vi "[BLE Test] ble_read_write_characteristics (old).vi"() -> ()   [LabVIEW 2015]
uses:
  Lib_Bled112 toolkit/type_def/connection_status_bundle.ctl
  Lib_Bled112 toolkit/type_def/address_type.ctl
  Lib_Bled112 toolkit/ble_functions/ble_write_by_service_characteristic_uint8array.vi
  Lib_Bled112 toolkit/ble_functions/ble_write_by_handle_uint8array.vi
panel:
  out "Scan success?":bool
  out "BLED112 Dongle Info":string="Major: 1, Minor: 3, Patch: 2, Build: 122, LL ver: 3, Protocol ver: 1 and HW ver: 3  "
  out "그래프 타이머 값 1":u32=9582380
  out "CDC(PCAP02) Graph":waveform(sgl)[](graph)=[{"t0"=timestamp(3554331896.4574084 s since 1904-01-01), "dt"=0.03, "Y"=[1.0007696]}, {"t0"=timestamp(3554331896.4574084 s since 1904-01-01), "dt"=0.03, "Y"=[1.0004687]}]
  out "Working Time(H:M:S)":string="00:01:58"
  out "ms 타이머 값 2":u32=9464045
  out "Get Device name":bool
  out "Get handle table":bool
  in  "Device List":i32(listbox)=2
  out "Rx packet Interval graph":u32(graph)=30
  in  "Program Exit":bool=TRUE
  in  "Set-Interval":bool
  out "Rx 2":bool=TRUE
  out "부분배열 2":u8[](array[numeric])=[253, 79, 255, 49, 255, 79, 255, 60, 255, 209, 65, 123, 0, 0, 0, 0, 0, 0, 0, 0] format="%x"
  out "Data-IMU":dbl=-3.014375 format="%.10f"
  out "Hex-IMU":i16=-689 format="%x"
  out "웨이브폼 차트-IMU":dbl(graph)=-3.014375
  in  "Index-IMU ch.":u8(slide)=1 min=1 max=6 step=1 scale=1.0..6.0
  out "Rx 문자열 2":string
  out "IMU-Rx time(ms)":u32=15
  out "IMU Rx OK":bool=TRUE
  out "CDC Rx OK":bool=TRUE
  out "CDC-Rx time(ms)":u32=15
  out "ms 타이머 값":u32=9582439
  out "Entire-Rx time(ms)":i32=30
  in  "Index-CDC ch.":u8(slide)=1 min=1 max=6 step=1 scale=1.0..6.0
  out "웨이브폼 차트 - CDC":sgl(graph)=1.0007696
  out "Hex-CDC":u32=2098766 format="%x"
  out "Data-CDC":dbl=1.0007696151733398 format="%.10f"
  out "부분배열":u8[](array[numeric])=[32, 6, 78, 32, 3, 215, 32, 6, 110, 32, 71, 249, 32, 115, 92, 32, 30, 38, 1, 0] format="%x"
  out "Rx 1":bool=TRUE
  in  "Tx 문자열":string="\nBLED112 Test\n"
  in  "Tx Send":bool
  out "Rx Cnt":i32=3775
  in  "Rx Stop":bool=TRUE
  out "Rx 문자열 1":string
  out "Connected":bool
  out "Device Name":string
  out "Address Type":enum16{"Public", "Random"}(ring)=enum."Random"
  out "Handle table":string[][](array[string])
  out "Connection Status":T1 {"Address Type" items=["Public", "Random"]}
  out "Scanning":bool
  in  "Device Connect":bool=TRUE
  out "MAC Address":string="D9:2F:10:92:34:F2"
  in  "COM Bluegiga in":refnum<visa-resource-name>="COM8"
  # "GEN4 1st PP - BLE(Bluetooth Low Energy) Test"
  # "CDC Data"
  # "SCAN"
  # "DEVICES FOUND"
  # "CONNECT"
  # "Introduce the MAC Address and Address Type of the device you want to connect and click in the CONTINUE button"
  # "IMU Data"
  # "Service 0x1800\nCharacteristic 0x2A00\nDevice Name"
  # "READING DEVICE NAME"
  # "Read"
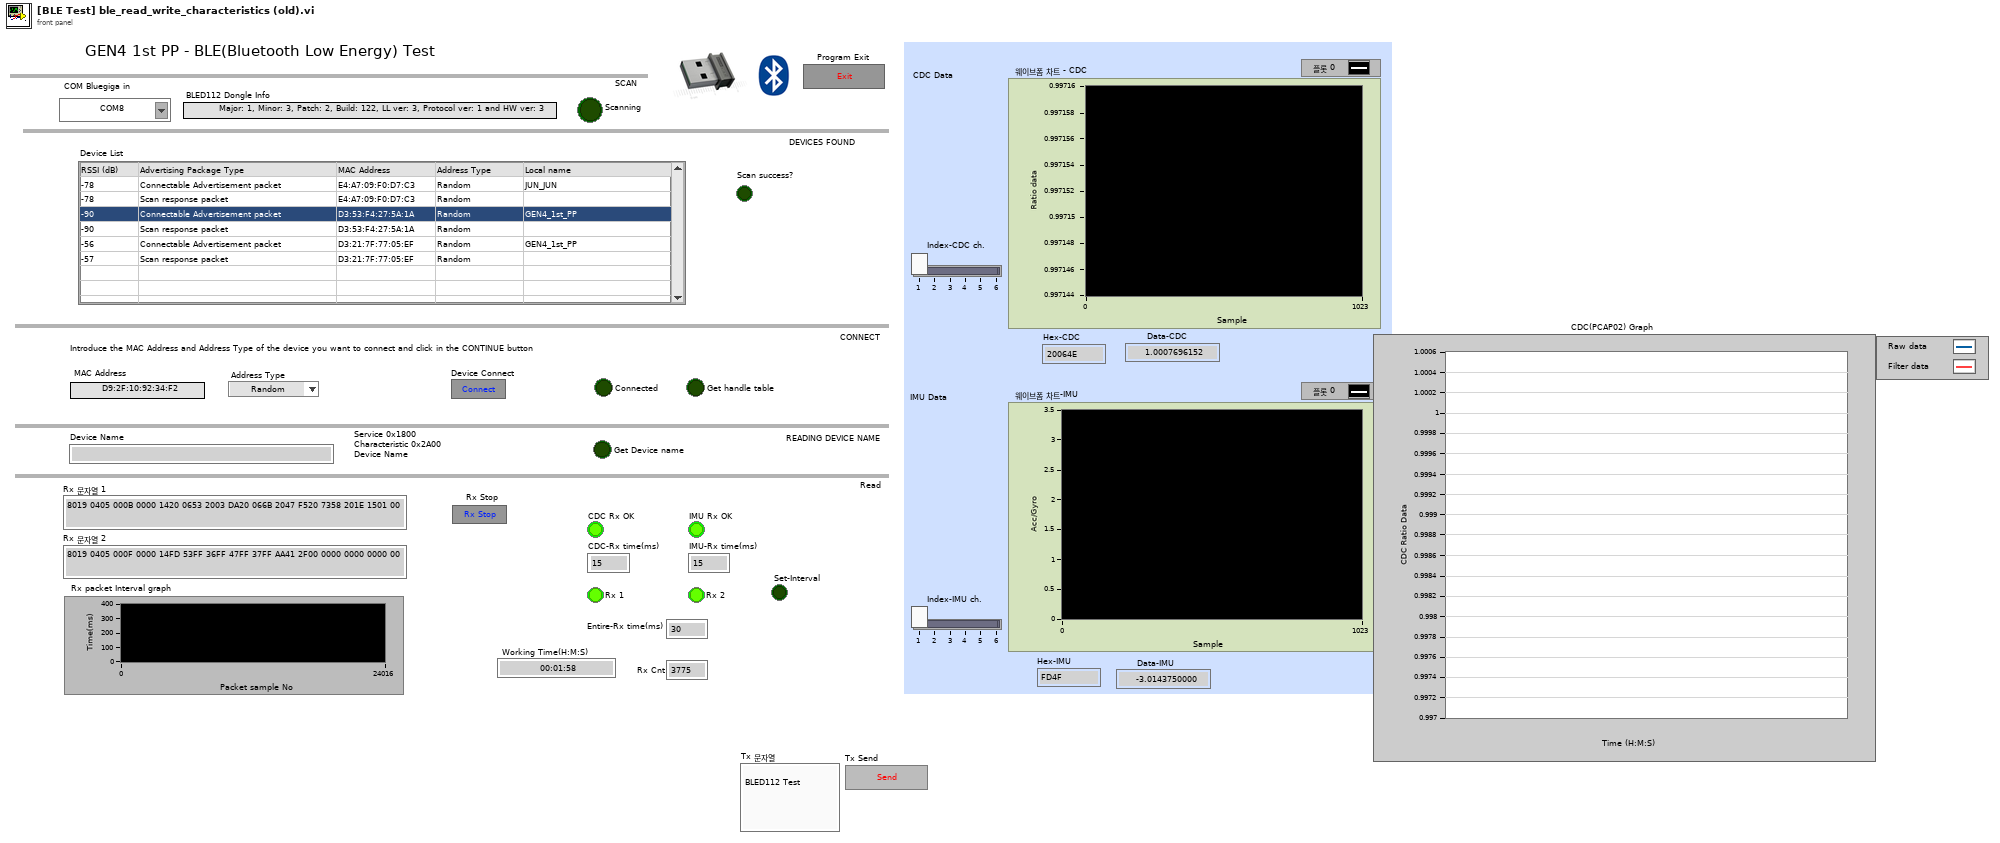
[diagram p1: front panel]
types:
  T1 = typedef "connection_status_bundle.ctl" = cluster{"MAC Address":string, "cnx handle":u8, "cnx flags":u8, "Address Type":T2, "Connection Interval (ms)":u16, "Timeout(ms)":u16, "Latency":u16, "bonding handle":u8}
  T2 = typedef "address_type.ctl" = u8
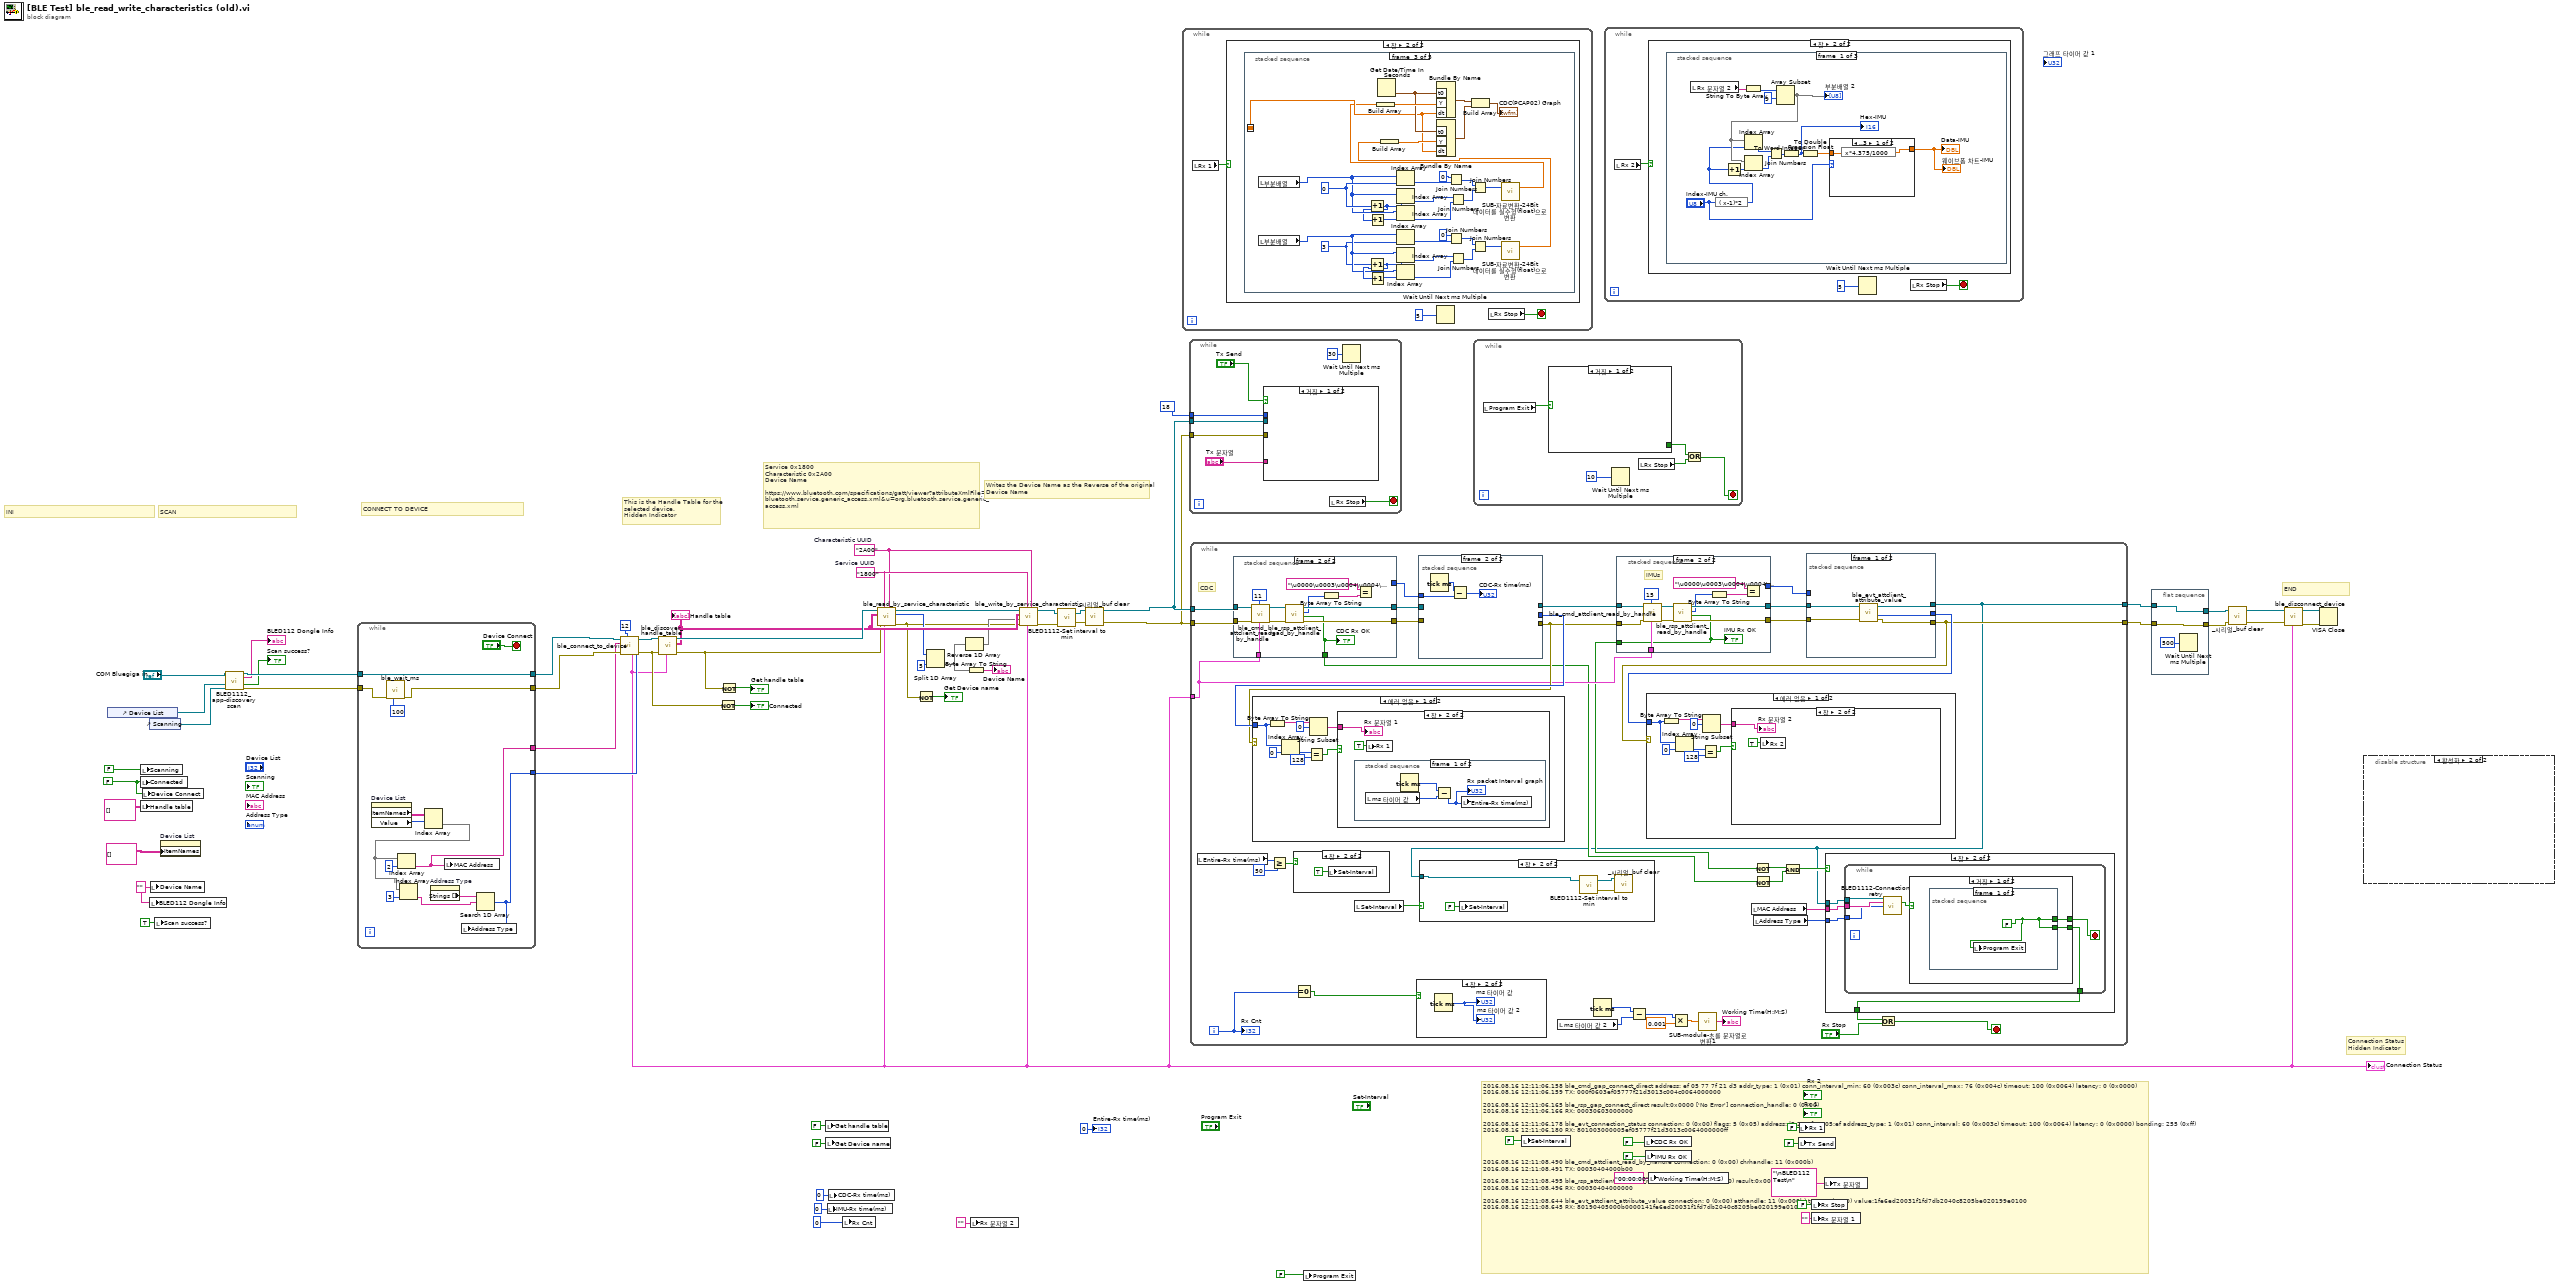
[diagram p0: block diagram]
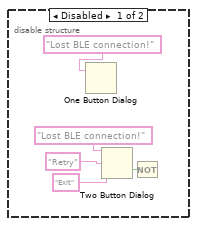
[diagram p2: hidden frame]
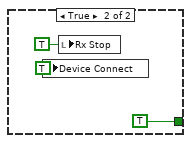
[diagram p3: hidden frame]
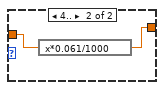
[diagram p5: hidden frame]
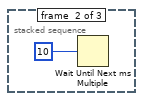
[diagram p6: hidden frame]
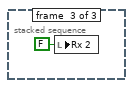
[diagram p7: hidden frame]
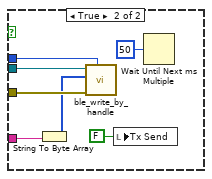
[diagram p8: hidden frame]
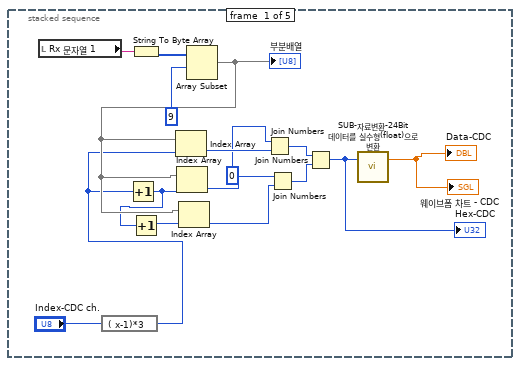
[diagram p10: hidden frame]
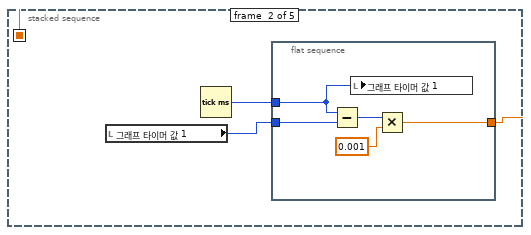
[diagram p11: hidden frame]
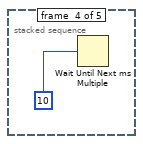
[diagram p12: hidden frame]
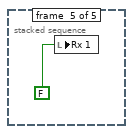
[diagram p13: hidden frame]
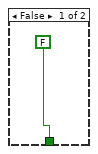
[diagram p16: hidden frame]
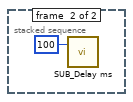
[diagram p17: hidden frame]
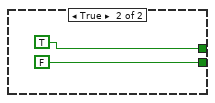
[diagram p18: hidden frame]
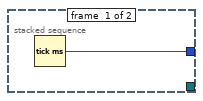
[diagram p20: hidden frame]
diagram:
  w50 = "2A00"  # Characteristic UUID
  w51 = "1800"  # Service UUID
  w4 = "" ("Device Name")
  w61 = FALSE ("Connected")
  # "2016.08.16 12:11:06.158 ble_cmd_gap_connect_direct address: ef 05 77 7f 21 d3 addr_type: 1 (0x01) conn_interval_min: 60 (0x003c) conn_interval_max: 76 (0x004c) timeout: 100 (0x0064) latency: 0 (0x0000)\n2016.08.16 12:11:06.159 TX: 000f0603ef05777f21d3013c004c0064000000\n\n2016.08.16 12:11:06.165 ble_rsp_gap_connect_direct result:0x0000 ['No Error'] connection_handle: 0 (0x00)\n2016.08.16 12:11:06.166 RX: 00030603000000\n\n2016.08.16 12:11:06.178 ble_evt_connection_status connection: 0 (0x00) flags: 5 (0x05) address:d3:21:7f:77:05:ef address_type: 1 (0x01) conn_interval: 60 (0x003c) timeout: 100 (0x0064) latency: 0 (0x0000) bonding: 255 (0xff)\n2016.08.16 12:11:06.180 RX: 801003000005ef05777f21d3013c0064000000ff\n\n\n\n\n2016.08.16 12:11:08.490 ble_cmd_attclient_read_by_handle connection: 0 (0x00) chrhandle: 11 (0x000b)\n2016.08.16 12:11:08.491 TX: 00030404000b00\n\n2016.08.16 12:11:08.495 ble_rsp_attclient_read_by_handle connection: 0 (0x00) result:0x0000 ['No Error']\n2016.08.16 12:11:08.496 RX: 00030404000000\n\n2016.08.16 12:11:08.644 ble_evt_attclient_attribute_value connection: 0 (0x00) atthandle: 11 (0x000b) type: 0 (0x00) value:1fe6ed20031f1fd7db2040c8205be020199e0100\n2016.08.16 12:11:08.645 RX: 80190405000b0000141fe6ed20031f1fd7db2040c8205be020199e0100"
  # "Writes the Device Name as the Reverse of the original\nDevice Name"
  # "Service 0x1800\nCharacteristic 0x2A00\nDevice Name\n\nhttps://www.bluetooth.com/specifications/gatt/viewer?attributeXmlFile=org.bluetooth.service.generic_access.xml&u=org.bluetooth.service.generic_access.xml"
  # "This is the Handle Table for the\nselected device. \nHidden Indicator"
  # "Connection Status\nHidden Indicator"
  # "CONNECT TO DEVICE"
  # "SCAN"
  # "END"
  # "INI"
  n1 = control-ref of="Device List"() -> (w8:refnum<vi>)
  n2 = local write "Connected"(w61) -> ()
  n3 = local write "Handle table"(string[][] [] ("Handle table")) -> ()
  n4 = local write "Scanning"(FALSE ("Scanning")) -> ()
  n5 = local write "Device Connect"(w61) -> ()
  n6 = control-ref of="Scanning"() -> (w7:refnum<vi>)
  n7 = local write "BLED112 Dongle Info"(w4) -> ()
  n8 = local write "Device Name"(w4) -> ()
  n9 = local write "Scan success?"(TRUE ("Scan success?")) -> ()
  n10 = property on="Device List" class="MCListbox (엄격한)"("ItemNames"=string[][] [] ("Devices")) -> ()  [unwired: 2 in, 2 out]
  n11 = call "BLED1112_app-discovery scan.vi"("COM in"="COM Bluegiga in", "Device List"=w8, "LED ref"=w7) -> ("COM out"=w6:refnum<visa-resource-name>, "BLED112 Dongle Info"=→"BLED112 Dongle Info":string, "Scan success?"=→"Scan success?":bool, "error out"=w3:errorcluster)  [unwired: 8 in, 1 out]
  n12 = while {
    tunnel: w3 -> [w81]
    tunnel: [w80] -> w68
    tunnel: w6 -> [w80]
    tunnel: [w79] -> w67
    tunnel: [w74] -> w64
    tunnel: [w69] -> w63
    stop <- "Device Connect" stop-if-true
    n13 = property on="Device List" class="MCListbox (엄격한)"() -> ("ItemNames"=w77:string[][], "Value"=w76:i32)  [unwired: 2 in, 2 out]
    n14 = call "ble_wait_ms.vi"("milliseconds to wait (100)"=u32 100, "error in (no error)"=w81) -> ("error out"=w79:errorcluster)  [unwired: 9 in]
    n15 = Index Array(array=w77, index (row)=w76) -> (element=w72:string[])  [unwired: 1 in]
    n16 = Index Array(array=w72, index=2 ("인덱스")) -> (element=w74:string)
    n17 = Index Array(array=w72, index=3 ("인덱스")) -> (element=w70:string)
    n18 = property on="Address Type" class="Enum (엄격한)"() -> ("Strings []"=w71:string[])  [unwired: 2 in, 2 out]
    n19 = local write "MAC Address"(w74) -> ()
    n20 = Search 1D Array(1D array=w71, element=w70) -> (index of element=w69:i32)  [unwired: 1 in]
    n21 = local write "Address Type"(w69) -> ()
  }
  n22 = call "ble_connect_to_device.vi"("Address Type"=w63, "Connection Interval Min (75ms)"=u16 12, "error in (no error)"=w67, "MAC Address"=w64, "COM Bluegiga in"=w68) -> ("error out"=w36:errorcluster, "COM Bluegiga out"=w38:refnum<visa-resource-name>, "Connection Status"=w14:T1)  [unwired: 4 in]
  "Connection Status" <- w14
  n23 = call "ble_discover_handle_table.vi"("Connection Status"=w14, "error in (no error)"=w36, "COM Bluegiga in"=w38) -> ("error out"=w35:errorcluster, "Handle table"=w49:string[][], "COM Bluegiga out"=w55:refnum<visa-resource-name>)  [unwired: 6 in]
  "Handle table" <- w49
  n24 = Not(x=w36) -> (.not. x?=→"Connected":bool)
  n25 = Not(x=w35) -> (.not. x?=→"Get handle table":bool)
  n26 = local write "Get handle table"(FALSE ("Get handle table")) -> ()
  n27 = local write "Get Device name"(FALSE ("Get Device name")) -> ()
  n28 = local write "IMU-Rx time(ms)"(u32 0 ("CDC-Rx time(ms)")) -> ()
  n29 = local write "CDC-Rx time(ms)"(u32 0 ("CDC-Rx time(ms)")) -> ()
  n30 = local write "Rx Cnt"(u32 0 ("CDC-Rx time(ms)")) -> ()
  n31 = call "ble_read_by_service_characteristic.vi"("Characteristic UUID"=w50, "Connection Status"=w14, "Service UUID"=w51, "error in (no error)"=w35, "Handle table"=w49, "COM Bluegiga in"=w55) -> ("error out"=w32:errorcluster, "characteristic value"=w48:u8[], "COM Bluegiga out"=w52:refnum<visa-resource-name>)  [unwired: 3 in]
  n32 = Not(x=w32) -> (.not. x?=→"Get Device name":bool)
  n33 = Split 1D Array(array=w48, index=5) -> (second subarray=w47:u8[])  [unwired: 1 out]
  n34 = Reverse 1D Array(array=w47) -> (reversed array=w46:u8[])
  n35 = Byte Array To String(unsigned byte array=w47) -> (string=→"Device Name":string)
  n36 = local write "Rx 문자열 2"("" ("Rx 문자열 2")) -> ()
  n37 = call-poly "ble_write_by_service_characteristic.vi"("Characteristic UUID"=w50, "Connection Status"=w14, "Service UUID"=w51, "error in (no error)"=w32, "data"=w46, "Handle table"=w49, "COM Bluegiga in"=w52) -> ("error out"=w24:errorcluster, "COM Bluegiga out"=w25:refnum<visa-resource-name>)  [unwired: 3 in]
  n38 = call "BLED1112-Set interval to min.vi"("에러 입력(에러 없음)"=w24, "VISA 리소스 이름"=w25) -> ("에러 출력"=w22:errorcluster, "VISA 리소스 이름 출력"=w23:refnum<visa-resource-name>)
  n39 = call "_시리얼_buf clear.vi"("에러 출력 2"=w22, "시리얼 포트"=w23) -> ("에러 출력"=w43:errorcluster, "시리얼 포트 2"=w44:refnum<visa-resource-name>)  [unwired: 2 in]
  n40 = while {
    stop <- w85 stop-if-true
    n41 = local read "Rx 1"() -> (w84:bool)
    n42 = case shown="참" w84 {
      frame False {
      }
      frame True {
        n43 = stacked-sequence {
          seq-local: [_ w102 _ _ _] -> [_ _ w134 _ _]
          frame #0 {
            n44 = local read "Rx 문자열 1"() -> (w101:string)
            n45 = expression code="( x-1)*3"("Index-CDC ch.") -> (w88:u8)
            n46 = Increment(x=w88) -> (x+1=w87:u8)
            n47 = String To Byte Array(string=w101) -> (unsigned byte array=w100:u8[])
            n48 = Increment(x=w87) -> (x+1=w86:u8)
            n49 = Array Subset(array=w100, index=9 ("인덱스")) -> (w98:u8[])  [unwired: 1 in]
            "부분배열" <- w98
            n50 = Index Array(array=w98, index=w88) -> (element=w95:u8)
            n51 = Index Array(array=w98, index=w87) -> (element=w96:u8)
            n52 = Index Array(array=w98, index=w86) -> (element=w97:u8)
            n53 = Join Numbers(hi=u8 0 ("인덱스"), lo=w95) -> ((hi.lo)=w92:u16)
            n54 = Join Numbers(hi=w96, lo=w97) -> ((hi.lo)=w93:u16)
            n55 = Join Numbers(hi=w92, lo=w93) -> ((hi.lo)=w91:u32)
            "Hex-CDC" <- w91
            n56 = call "SUB-자료변환-24Bit 데이터를 실수형(float)으로 변환.vi"("U32"=w91) -> ("FP32"=→"Data-CDC" →"웨이브폼 차트 - CDC":sgl)  [unwired: 2 in]
          }
          frame #1 {
            n57 = local read "그래프 타이머 값 1"() -> (w104:u32)
            n58 = Tick Count (ms)() -> (millisecond timer value=w103:u32)
            n59 = flat-sequence {
              tunnel: w103 -> [w109]
              tunnel: w104 -> [w106]
              tunnel: [w105] -> w102
              frame #0 {
                n60 = Subtract(x=w109, y=w106) -> (x-y=w107:u32)
                n61 = local write "그래프 타이머 값 1"(w109) -> ()
                n62 = Multiply(x=w107, y=0.001 ("dt")) -> (x*y=w105:dbl)
              }
            }
          }
          frame #2 {
            w112 = u8 3 ("인덱스")
            w133 = u8 0 ("인덱스")
            n63 = local read "부분배열"() -> (w132:u8[])
            n64 = local read "부분배열"() -> (w113:u8[])
            n65 = Increment(x=w133) -> (x+1=w124:u8)
            n66 = Increment(x=w112) -> (x+1=w121:u8)
            n67 = Increment(x=w124) -> (x+1=w123:u8)
            n68 = Increment(x=w121) -> (x+1=w122:u8)
            n69 = Get Date/Time In Seconds() -> (seconds since 1Jan1904=w138:timestamp)
            n70 = Index Array(array=w132, index=w133) -> (element=w129:u8)
            n71 = Index Array(array=w113, index=w112) -> (element=w116:u8)
            n72 = Index Array(array=w132, index=w124) -> (element=w130:u8)
            n73 = Index Array(array=w132, index=w123) -> (element=w131:u8)
            n74 = Index Array(array=w113, index=w121) -> (element=w115:u8)
            n75 = Index Array(array=w113, index=w122) -> (element=w114:u8)
            n76 = Join Numbers(hi=u8 0 ("인덱스"), lo=w129) -> ((hi.lo)=w126:u16)
            n77 = Join Numbers(hi=u8 0 ("인덱스"), lo=w116) -> ((hi.lo)=w119:u16)
            n78 = Join Numbers(hi=w130, lo=w131) -> ((hi.lo)=w127:u16)
            n79 = Join Numbers(hi=w115, lo=w114) -> ((hi.lo)=w118:u16)
            n80 = Join Numbers(hi=w126, lo=w127) -> ((hi.lo)=w125:u32)
            n81 = Join Numbers(hi=w119, lo=w118) -> ((hi.lo)=w120:u32)
            n82 = call "SUB-자료변환-24Bit 데이터를 실수형(float)으로 변환.vi"("U32"=w125) -> ("FP32"=w111:sgl)  [unwired: 2 in]
            n83 = Build Array(w111) -> (w139:sgl[])
            n84 = Bundle By Name("t0"=w138, "Y"=w139, "dt"=w134) -> (w135:waveform(sgl))  [unwired: 1 in]
            n85 = call "SUB-자료변환-24Bit 데이터를 실수형(float)으로 변환.vi"("U32"=w120) -> ("FP32"=w110:sgl)  [unwired: 2 in]
            n86 = Build Array(w110) -> (w140:sgl[])
            n87 = Bundle By Name("t0"=w138, "Y"=w140, "dt"=w134) -> (w136:waveform(sgl))  [unwired: 1 in]
            n88 = Build Array(w135, w136) -> (→"CDC(PCAP02) Graph":waveform(sgl)[])
          }
          frame #3 {
            n89 = Wait Until Next ms Multiple(millisecond multiple=u32 10 ("ms 배수")) -> ()  [unwired: 1 out]
          }
          frame #4 {
            n90 = local write "Rx 1"(FALSE ("Rx")) -> ()
          }
        }
      }
    }
    n91 = Wait Until Next ms Multiple(millisecond multiple=u32 5 ("ms 배수")) -> ()  [unwired: 1 out]
    n92 = local read "Rx Stop"() -> (w85:bool)
  }
  n93 = while {
    tunnel: w44 -> [w146]
    tunnel: w43 -> [w145]
    tunnel: u16 18 ("Handle") -> [w144]
    stop <- w147 stop-if-true
    n94 = case shown="거짓" "Tx Send" {
      tunnel: w146 -> [_ w156]
      tunnel: w145 -> [_ w155]
      tunnel: w144 -> [_ w153]
      tunnel: "Tx 문자열" -> [_ w152]
      frame False {
      }
      frame True {
        n95 = String To Byte Array(string=w152) -> (unsigned byte array=w154:u8[])
        n96 = call-poly "ble_write_by_handle.vi"("Handle"=w153, "error in (no error)"=w155, "data (uint8array)"=w154, "COM Bluegiga in"=w156) -> ()  [unwired: 6 in, 2 out]
        n97 = local write "Tx Send"(FALSE ("Tx Send")) -> ()
        n98 = Wait Until Next ms Multiple(millisecond multiple=u32 50 ("ms 배수")) -> ()  [unwired: 1 out]
      }
    }
    n99 = local read "Rx Stop"() -> (w147:bool)
    n100 = Wait Until Next ms Multiple(millisecond multiple=u32 30 ("ms 배수")) -> ()  [unwired: 1 out]
  }
  n101 = while {
    tunnel: w44 -> [w190]
    tunnel: w43 -> [w189]
    tunnel: w14 -> [w184]
    tunnel: [w160] -> w59
    tunnel: [w182] -> w58
    i -> [w168]
    stop <- w176 stop-if-true
    # "CDC"
    n102 = local read "Entire-Rx time(ms)"() -> (w171:i32)
    n103 = stacked-sequence {
      tunnel: [_ w239] -> w192
      tunnel: [_ w238] -> w191
      tunnel: w190 -> [_ w237]
      tunnel: w189 -> [_ w236]
      tunnel: w184 -> [_ w235]
      tunnel: [w230 _] -> w181
      tunnel: [_ w231] -> w173
      frame #0 {
        n104 = Tick Count (ms)() -> (millisecond timer value=w230:u32)
      }
      frame #1 {
        n105 = call "ble_cmd_attclient_read_by_handle.vi"("Connection Status"=w235, "chrHandle"=u16 11 ("Handle"), "error in (no error)"=w236, "COM Bluegiga in"=w237) -> ("error out"=w240:errorcluster, "COM Bluegiga out"=w241:refnum<visa-resource-name>)  [unwired: 6 in]
        n106 = call "ble_rsp_attclient_read_by_handle.vi"("error in (no error)"=w240, "COM Bluegiga in"=w241) -> ("error out"=w239:errorcluster, "success?"=w231:bool, "full message package"=w232:u8[], "COM Bluegiga out"=w238:refnum<visa-resource-name>)  [unwired: 6 in]
        "CDC Rx OK" <- w231
        n107 = Byte Array To String(unsigned byte array=w232) -> (string=w233:string)
        n108 = Equal?(x="\u0000\u0003\u0004\u0004\u0000\u0000\u0000", y=w233) -> ()  [unwired: 1 out]
      }
    }
    n109 = Greater Or Equal?(x=w171, y=50) -> (x >= y?=w170:bool)
    n110 = case shown="참" w170 {
      frame False {
      }
      frame True {
        n111 = local write "Set-Interval"(TRUE ("Set-Interval")) -> ()
      }
    }
    n112 = Equal To 0?(x=w168) -> (x = 0?=w167:bool)
    n113 = local read "Set-Interval"() -> (w179:bool)
    n114 = case shown="참" w167 {
      frame False {
      }
      frame True {
        n115 = Tick Count (ms)() -> (millisecond timer value=→"ms 타이머 값" →"ms 타이머 값 2":u32)
      }
    }
    n116 = stacked-sequence {
      tunnel: [w263 _] -> w186
      tunnel: [w261 _] -> w193
      tunnel: [w262 _] -> w185
      tunnel: w192 -> [w265 _]
      tunnel: w191 -> [w264 _]
      tunnel: w181 -> [_ w267]
      frame #0 {
        n117 = call "ble_evt_attclient_attribute_value.vi"("error in (no error)"=w265, "COM Bluegiga in"=w264) -> ("error out"=w262:errorcluster, "full message package"=w261:u8[], "COM Bluegiga out"=w263:refnum<visa-resource-name>)  [unwired: 6 in, 1 out]
      }
      frame #1 {
        n118 = Tick Count (ms)() -> (millisecond timer value=w268:u32)
        n119 = Subtract(x=w268, y=w267) -> (x-y=→"CDC-Rx time(ms)":u32)
      }
    }
    n120 = case shown="에러 없음" w185 {
      tunnel: w193 -> [w274 _]
      frame No Error {
        n121 = Byte Array To String(unsigned byte array=w274) -> (string=w276:string)
        n122 = Index Array(array=w274, index=0 ("인덱스")) -> (element=w272:u8)
        n123 = Equal?(x=w272, y=u16 128 ("Handle")) -> (x = y?=w270:bool)
        n124 = String Subset(string=w276, offset (0)=0 ("오프셋(0)")) -> (substring=w269:string)  [unwired: 1 in]
        n125 = case shown="참" w270 {
          tunnel: w269 -> [_ w278]
          frame False {
          }
          frame True {
            n126 = stacked-sequence {
              frame #0 {
                n127 = local read "ms 타이머 값"() -> (w281:u32)
                n128 = Tick Count (ms)() -> (millisecond timer value=w280:u32)
                n129 = Subtract(x=w280, y=w281) -> (x-y=w279:u32)
                "Rx packet Interval graph" <- w279
                n130 = local write "Entire-Rx time(ms)"(w279) -> ()
              }
              frame #1 {
                n131 = Tick Count (ms)() -> (millisecond timer value=w282:u32)
                n132 = local write "ms 타이머 값"(w282) -> ()
              }
            }
            n133 = local write "Rx 1"(TRUE ("Rx")) -> ()
            "Rx 문자열 1" <- w278
          }
        }
      }
      frame Error {
      }
    }
    n134 = local read "ms 타이머 값 2"() -> (w165:u32)
    n135 = Tick Count (ms)() -> (millisecond timer value=w166:u32)
    n136 = stacked-sequence {
      tunnel: [_ w229] -> w188
      tunnel: [_ w228] -> w187
      tunnel: w186 -> [_ w224]
      tunnel: w185 -> [_ w223]
      tunnel: w184 -> [_ w222]
      tunnel: [w217 _] -> w180
      tunnel: [_ w218] -> w172
      frame #0 {
        n137 = Tick Count (ms)() -> (millisecond timer value=w217:u32)
      }
      frame #1 {
        # "IMUs"
        n138 = call "ble_cmd_attclient_read_by_handle.vi"("Connection Status"=w222, "chrHandle"=u16 15 ("Handle"), "error in (no error)"=w223, "COM Bluegiga in"=w224) -> ("error out"=w227:errorcluster, "COM Bluegiga out"=w226:refnum<visa-resource-name>)  [unwired: 6 in]
        n139 = call "ble_rsp_attclient_read_by_handle.vi"("error in (no error)"=w227, "COM Bluegiga in"=w226) -> ("error out"=w228:errorcluster, "success?"=w218:bool, "full message package"=w219:u8[], "COM Bluegiga out"=w229:refnum<visa-resource-name>)  [unwired: 6 in]
        "IMU Rx OK" <- w218
        n140 = Byte Array To String(unsigned byte array=w219) -> (string=w220:string)
        n141 = Equal?(x="\u0000\u0003\u0004\u0004\u0000\u0000\u0000", y=w220) -> ()  [unwired: 1 out]
      }
    }
    n142 = Subtract(x=w166, y=w165) -> (x-y=w162:u32)
    n143 = Multiply(x=w162, y=0.001) -> (x*y=w164:dbl)
    n144 = call "SUB-module-초를 문자열로 변환1.vi"("입력-초단위"=w164) -> ("시:분:초"=→"Working Time(H:M:S)":string)
    n145 = local read "MAC Address"() -> (w158:string)
    n146 = local read "Address Type"() -> (w157:enum16{"Public", "Random"})
    n147 = Not(x=w172) -> (.not. x?=w174:bool)
    n148 = Not(x=w173) -> (.not. x?=w175:bool)
    n149 = And(x=w174, y=w175) -> (x .and. y?=w177:bool)
    n150 = stacked-sequence {
      tunnel: [w255 _] -> w160
      tunnel: [w253 _] -> w183
      tunnel: [w254 _] -> w182
      tunnel: w187 -> [w257 _]
      tunnel: w188 -> [w256 _]
      tunnel: w180 -> [_ w259]
      frame #0 {
        n151 = call "ble_evt_attclient_attribute_value.vi"("error in (no error)"=w257, "COM Bluegiga in"=w256) -> ("error out"=w254:errorcluster, "full message package"=w253:u8[], "COM Bluegiga out"=w255:refnum<visa-resource-name>)  [unwired: 6 in, 1 out]
      }
      frame #1 {
        n152 = Tick Count (ms)() -> (millisecond timer value=w260:u32)
        n153 = Subtract(x=w260, y=w259) -> (x-y=→"IMU-Rx time(ms)":u32)
      }
    }
    n154 = case shown="참" w179 {
      tunnel: w160 -> [_ w213]
      frame False {
      }
      frame True {
        n155 = local write "Set-Interval"(FALSE ("Set-Interval")) -> ()
        n156 = call "BLED1112-Set interval to min.vi"("VISA 리소스 이름"=w213) -> ("에러 출력"=w214:errorcluster, "VISA 리소스 이름 출력"=w215:refnum<visa-resource-name>)  [unwired: 1 in]
        n157 = call "_시리얼_buf clear.vi"("에러 출력 2"=w214, "시리얼 포트"=w215) -> ()  [unwired: 2 in, 2 out]
      }
    }
    n158 = case shown="에러 없음" w182 {
      tunnel: w183 -> [w248 _]
      frame No Error {
        n159 = Byte Array To String(unsigned byte array=w248) -> (string=w250:string)
        n160 = Index Array(array=w248, index=0 ("인덱스")) -> (element=w246:u8)
        n161 = Equal?(x=w246, y=u16 128 ("Handle")) -> (x = y?=w244:bool)
        n162 = String Subset(string=w250, offset (0)=0 ("오프셋(0)")) -> (substring=w243:string)  [unwired: 1 in]
        n163 = case shown="참" w244 {
          tunnel: w243 -> [_ w252]
          frame False {
          }
          frame True {
            n164 = local write "Rx 2"(TRUE ("Rx")) -> ()
            "Rx 문자열 2" <- w252
          }
        }
      }
      frame Error {
      }
    }
    n165 = case shown="참" w177 {
      tunnel: w160 -> [_ w200]
      tunnel: [FALSE w197] -> w159
      tunnel: w158 -> [_ w199]
      tunnel: w157 -> [_ w198]
      frame False {
      }
      frame True {
        n166 = while {
          tunnel: w200 -> [w206]
          tunnel: w199 -> [w205]
          tunnel: w198 -> [w204]
          tunnel: [w201] -> w197
          stop <- w202 stop-if-true
          n167 = call "BLED1112-Connection retry.vi"("VISA 리소스 이름"=w206, "MAC Address"=w205, "Address Type"=w204) -> ("Connected"=w203:bool)  [unwired: 10 in, 2 out]
          n168 = case shown="거짓" w203 {
            tunnel: [w208 TRUE] -> w202
            tunnel: [w207 FALSE] -> w201
            frame False {
              n169 = stacked-sequence {
                tunnel: [w209 _] -> w208
                tunnel: [w209 _] -> w207
                frame #0 {
                  w209 = FALSE
                  n170 = local write "Program Exit"(w209) -> ()
                }
                frame #1 {
                  n171 = call "SUB_Delay ms.vi"("delay(ms)"=u32 100) -> ()  [unwired: 3 in]
                }
              }
            }
            frame True {
            }
          }
        }
      }
    }
    n172 = Or(x=w159, y="Rx Stop") -> (x .or. y?=w176:bool)
    "Rx Cnt" <- w168
  }
  n173 = local write "Program Exit"(FALSE ("정지")) -> ()
  n174 = while {
    stop <- w283 stop-if-true
    n175 = local read "Program Exit"() -> (w287:bool)
    n176 = case shown="거짓" w287 {
      tunnel: [_ TRUE] -> w284
      frame False {
      }
      frame True {
        n177 = local write "Device Connect"(TRUE ("Continue")) -> ()
        n178 = local write "Rx Stop"(TRUE ("Rx 정지")) -> ()
      }
    }
    n179 = Wait Until Next ms Multiple(millisecond multiple=u32 10 ("ms 배수")) -> ()  [unwired: 1 out]
    n180 = local read "Rx Stop"() -> (w285:bool)
    n181 = Or(x=w284, y=w285) -> (x .or. y?=w283:bool)
  }
  n182 = local write "Set-Interval"(FALSE ("Set-Interval")) -> ()
  n183 = while {
    stop <- w293 stop-if-true
    n184 = local read "Rx 2"() -> (w292:bool)
    n185 = case shown="참" w292 {
      frame False {
      }
      frame True {
        n186 = stacked-sequence {
          frame #0 {
            n187 = local read "Rx 문자열 2"() -> (w306:string)
            n188 = expression code="( x-1)*2"("Index-IMU ch.") -> (w297:u8)
            n189 = Increment(x=w297) -> (x+1=w296:u8)
            n190 = String To Byte Array(string=w306) -> (unsigned byte array=w305:u8[])
            n191 = Array Subset(array=w305, index=9 ("인덱스")) -> (w303:u8[])  [unwired: 1 in]
            "부분배열 2" <- w303
            n192 = Index Array(array=w303, index=w297) -> (element=w302:u8)
            n193 = Index Array(array=w303, index=w296) -> (element=w301:u8)
            n194 = Join Numbers(hi=w302, lo=w301) -> ((hi.lo)=w299:u16)
            n195 = To Word Integer(number=w299) -> (16bit integer=w295:i16)
            "Hex-IMU" <- w295
            n196 = To Double Precision Float(number=w295) -> (double precision float=w298:dbl)
            n197 = case shown="..3" "Index-IMU ch." {
              tunnel: [w308 w309] -> w300
              tunnel: w298 -> [w307 w310]
              frame ..3 {
                n198 = expression code="x*4.375/1000"(w307) -> (w308:dbl)
              }
              frame 4.. {
                n199 = expression code="x*0.061/1000"(w310) -> (w309:dbl)
              }
            }
            "Data-IMU" <- w300
            "웨이브폼 차트-IMU" <- w300
          }
          frame #1 {
            n200 = Wait Until Next ms Multiple(millisecond multiple=u32 10 ("ms 배수")) -> ()  [unwired: 1 out]
          }
          frame #2 {
            n201 = local write "Rx 2"(FALSE ("Rx")) -> ()
          }
        }
      }
    }
    n202 = Wait Until Next ms Multiple(millisecond multiple=u32 5 ("ms 배수")) -> ()  [unwired: 1 out]
    n203 = local read "Rx Stop"() -> (w293:bool)
  }
  n204 = local write "CDC Rx OK"(FALSE ("success?")) -> ()
  n205 = local write "IMU Rx OK"(FALSE ("success?")) -> ()
  n206 = local write "Working Time(H:M:S)"("00:00:00" ("Working Time(H:M:S)")) -> ()
  n207 = local write "Tx Send"(FALSE ("Tx Send")) -> ()
  n208 = local write "Rx 1"(FALSE ("Rx")) -> ()
  n209 = local write "Rx Stop"(FALSE ("Rx 정지")) -> ()
  n210 = local write "Rx 문자열 1"("" ("Rx 문자열")) -> ()
  n211 = local write "Tx 문자열"("\nBLED112 Test\n" ("Tx 문자열")) -> ()
  n212 = flat-sequence {
    tunnel: [w314] -> w13
    tunnel: w59 -> [w314]
    tunnel: [w313] -> w12
    tunnel: w58 -> [w313]
    frame #0 {
      n213 = Wait Until Next ms Multiple(millisecond multiple=u32 500 ("ms 배수")) -> ()  [unwired: 1 out]
    }
  }
  n214 = call "_시리얼_buf clear.vi"("에러 출력 2"=w12, "시리얼 포트"=w13) -> ("에러 출력"=w11:errorcluster, "시리얼 포트 2"=w10:refnum<visa-resource-name>)  [unwired: 2 in]
  n215 = call "ble_disconnect_device.vi"("Connection Status"=w14, "error in (no error)"=w11, "COM Bluegiga in"=w10) -> ("error out"=w65:errorcluster, "COM Bluegiga out"=w66:refnum<visa-resource-name>)  [unwired: 7 in]
  n216 = VISA Close(VISA resource name=w66, error in (no error)=w65) -> ()  [unwired: 1 out]
  n217 = disable-structure shown="활성화" {
    frame Disabled {
      n218 = One Button Dialog(message="Lost BLE connection!" ("메시지")) -> ()  [unwired: 1 in, 1 out]
      n219 = Two Button Dialog(message="Lost BLE connection!" ("메시지"), 1:"Exit" ("참 버튼 이름(\"확인\")"), 2:"Retry" ("참 버튼 이름(\"확인\")")) -> (T button?=w319:bool)
      n220 = Not(x=w319) -> ()  [unwired: 1 out]
    }
    frame Enabled {
    }
  }
  "Entire-Rx time(ms)" <- 0 ("수신 주기(ms)")
